vi "Get ring selector waveform.vi"(7 "Clip/desimate":T1={"Clip time"=FALSE, "Tiime 0"=0.0, "Time 1"=0.0, "Maximum data points"=1, "Decimation method"=enum."Min-Max"}, 8 "Error In":errorcluster, 10 "Channel":u16(ring) items=["Select channel...", "Time", "Y"], 11 "File-group-channel":T2(array[cluster])) -> (0 "Error Out":errorcluster, 2 "Empty waveform":bool, 3 "Waveform":waveform(dbl))   [LabVIEW 2015]
uses:
  Controls/Data reduction.ctl
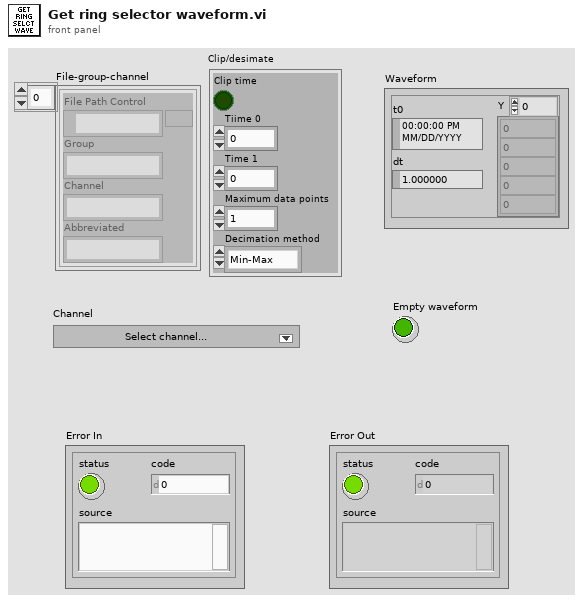
[diagram p1: front panel]
types:
  T1 = typedef "Data reduction.ctl" = cluster{"Clip time":bool, "Tiime 0":dbl, "Time 1":dbl, "Maximum data points":i32, "Decimation method":enum16{"coerce", "linear", "spline", "Min-Max", "Average"}}
  T2 = cluster{"File Path Control":path, "Group":string, "Channel":string, "Abbreviated":string}[]
  T3 = enum16{"open", "open or create", "create or replace", "create", "open (read-only)"}
  T4 = cluster{"File Path Control":path, "Group":string, "Channel":string, "Abbreviated":string}
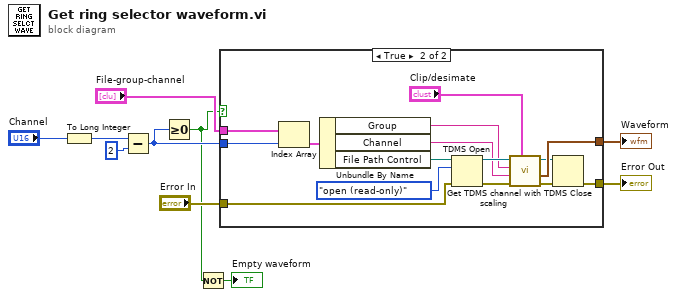
[diagram p0: block diagram]
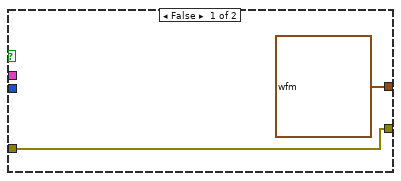
[diagram p2: hidden frame]
diagram:
  n1 = To Long Integer(number="Channel") -> (32bit integer=w5:i32)
  n2 = Subtract(x=w5, y=2) -> (x-y=w3:i32)
  n3 = Greater Or Equal To 0?(x=w3) -> (x >= 0?=w2:bool)
  n4 = Not(x=w2) -> (.not. x?=→"Empty waveform":bool)
  n5 = case shown="True" w2 {
    tunnel: w3 -> [_ w27]
    tunnel: [waveform(dbl) {"t0"=timestamp(0 s since 1904-01-01), "dt"=1.0, "Y"=[]} ("output waveform") w20] -> w7
    tunnel: "File-group-channel" -> [_ w19]
    tunnel: "Error In" -> [w11 w15]
    tunnel: [w11 w14] -> w8
    frame False {
    }
    frame True {
      n6 = Index Array(array=w19, index=w27) -> (element=w25:T4)
      n7 = Unbundle By Name(w25) -> ("Group"=w22:string, "Channel"=w21:string, "File Path Control"=w24:path)
      n8 = TDMS Open(8:w15, 10:T3."open (read-only)" ("operation (0:open)"), 11:w24) -> (0:w16:errorcluster, 3:w23:refnum<k34>)  [unwired: 4 in]
      n9 = call "Get TDMS channel with scaling.vi"("Clip/desimate"="Clip/desimate", "error in"=w16, "Channel name"=w21, "group name"=w22, "tdms file"=w23) -> ("error out"=w17:errorcluster, "output waveform"=w20:waveform(dbl), "tdms file out"=w18:refnum<k34>)  [unwired: 4 in]
      n10 = TDMS Close(8:w17, 11:w18) -> (0:w14:errorcluster)  [unwired: 1 out]
    }
  }
  "Error Out" <- w8
  "Waveform" <- w7
